vi "Brass_2.vi"(0 "Amount":fxp<+,8,0>, 4 "S/R":fxp<+,16,0>, 5 "1/Decay":fxp<+,16,0>, 6 "Sustain":fxp<+,16,0>, 7 "1/Attack":fxp<+,16,0>, 8 "Gate":bool, 10 "M":fxp<+,32,32>, 11 "Trigger":bool) -> (3 "Brass Out":fxp<+/-,8,8>)   [LabVIEW 2015]
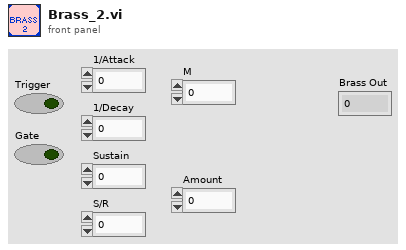
[diagram p1: front panel]
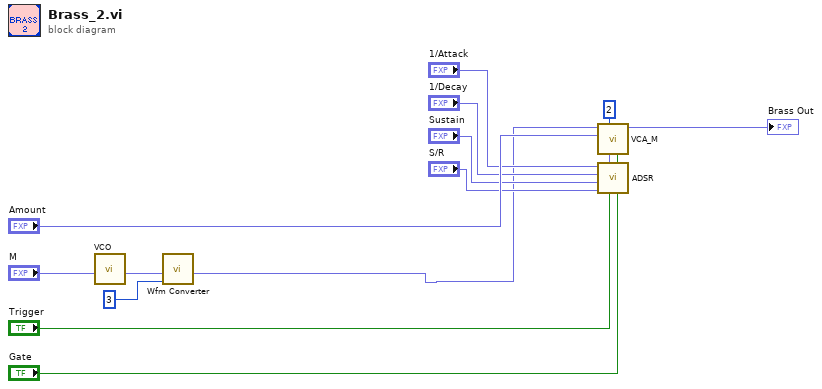
[diagram p0: block diagram]
diagram:
  n1 = call "VCO.vi"("M"="M") -> ("Sine Sample"=w5:fxp<+/-,8,8>)  [unwired: 10 in]
  n2 = call "Wfm Converter.vi"("Select"=u8 3 ("select"), "Sample In"=w5) -> ("Sample Out"=w1:fxp<+/-,8,8>)  [unwired: 9 in]
  n3 = call "ADSR.vi"("Gate"="Gate", "Trigger"="Trigger", "S/R"="S/R", "Sustain"="Sustain", "1/Decay"="1/Decay", "1/Attack"="1/Attack") -> ("Amount?"=w12:bool, "Sample Out"=w11:fxp<+,8,0>)  [unwired: 4 in]
  n4 = call "VCA_M.vi"("Amount?"=w12, "EG"=w11, "Scale"=i8 2, "Amount"="Amount", "Sample In"=w1) -> ("Sample Out"=→"Brass Out":fxp<+/-,8,8>)  [unwired: 6 in]
